vi "Channel_Control_Ramp.vi"(7 "Ramp Time / s":dbl=1.0 format="%0.2f", 8 "Error In":errorcluster, 10 "Aquisition rate/ Hz":dbl=20000.0 format="%0.2f", 11 "Output Chnnel Ramp":tag) -> (0 "Error Out":errorcluster, 3 "WRITE RAMP":refnum<k21>)   [LabVIEW 2023]
uses:
  <vilib>/DAQmx/create/channels.llb/DAQmx Create Channel (AO-Voltage-Basic).vi
  <vilib>/DAQmx/configure/timing.llb/DAQmx Timing (Sample Clock).vi
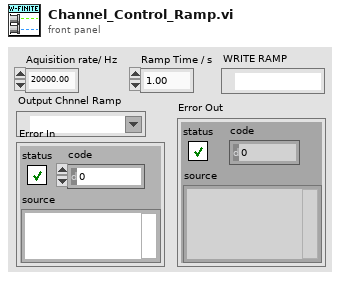
[diagram p1: front panel]
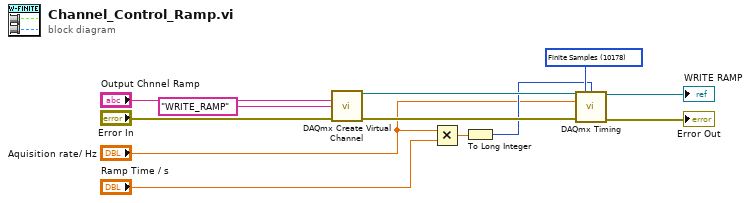
[diagram p0: block diagram]
diagram:
  w11 = 10178 items=["Finite Samples"=10178, "Continuous Samples"=10123, "Hardware Timed Single Point"=12522] ("sample mode")
  n1 = call-poly <vilib>:"DAQmx Create Virtual Channel.vi"("physical channels"="Output Chnnel Ramp", "name to assign"="WRITE_RAMP", "error in"="Error In") -> ("task out"=w9:refnum<k21>, "error out"=w7:errorcluster)  [unwired: 11 in]
  n2 = Multiply(x="Aquisition rate/ Hz", y="Ramp Time / s") -> (x*y=w3:dbl)
  n3 = To Long Integer(number=w3) -> (32bit integer=w6:i32)
  n4 = call-poly <vilib>:"DAQmx Timing.vi"("task/channels in"=w9, "sample mode"=w11, "samples per channel"=w6, "rate"="Aquisition rate/ Hz", "error in"=w7) -> ("task out"=→"WRITE RAMP":refnum<k21>, "error out"=→"Error Out":errorcluster)  [unwired: 9 in]
